vi "Data Type Enum to Data Type String.vi"(1 "data type":T1) -> (0 "format string":T2)   [LabVIEW 2019, in "LV-Data.PGSQL.lvclass"]
uses:
  LV-Data.PGSQL.lvclass
  Typedefs/Datatypes--combo.ctl
  Typedefs/Datatypes--enum.ctl
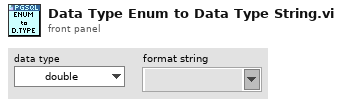
[diagram p1: front panel]
types:
  T1 = typedef "LV-Data.PGSQL.lvclass/Datatypes--enum.ctl" = enum16{"double", "string", "json", "integer", "boolean"}
  T2 = typedef "LV-Data.PGSQL.lvclass/Datatypes--combo.ctl" = string
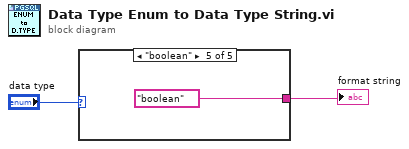
[diagram p0: block diagram]
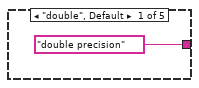
[diagram p2: hidden frame]
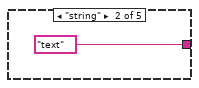
[diagram p3: hidden frame]
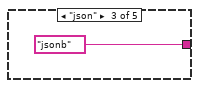
[diagram p4: hidden frame]
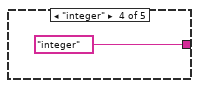
[diagram p5: hidden frame]
diagram:
  n1 = case shown="\"boolean\"" "data type" {
    tunnel: [T2 "double precision" ("new column data type") T2 "text" ("new column data type") T2 "jsonb" ("new column data type") T2 "integer" ("new column data type") T2 "boolean" ("new column data type")] -> w2
    frame "double", Default {
    }
    frame "string" {
    }
    frame "json" {
    }
    frame "integer" {
    }
    frame "boolean" {
    }
  }
  "format string" <- w2
